vi "Capture@ImageSave__Parameter.vi"(1 "ParamterIn":string) -> (0 "ParamterOut":string)   [LabVIEW 2020]
uses:
  MainFrame/Global.vi
panel:
  in  "Message":string(combo)
  out "Image":T1(plugin-control)
  in  "Picture":string(combo)
  in  "CamName":string(combo)
  in  "Confirm":bool
  # "Capture@General $Capture,$Picture(,[[$label]]$Message)"
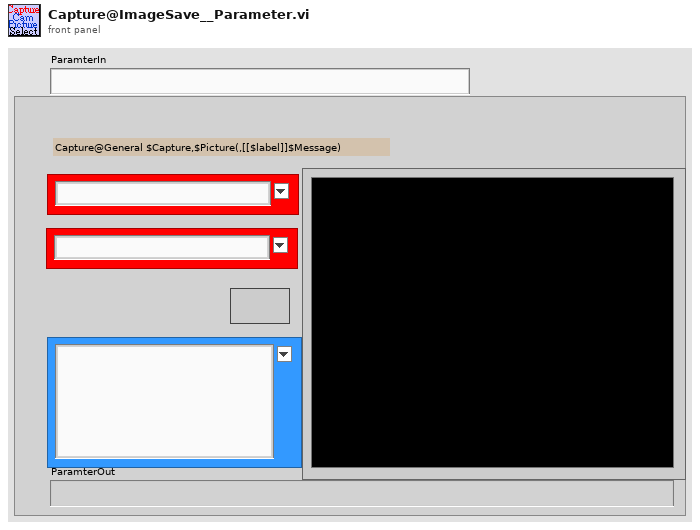
[diagram p1: front panel]
types:
  T1 = typedef "IMAQ Image.ctl" = refnum<image>
  T2 = typedef "Image Type" = u32
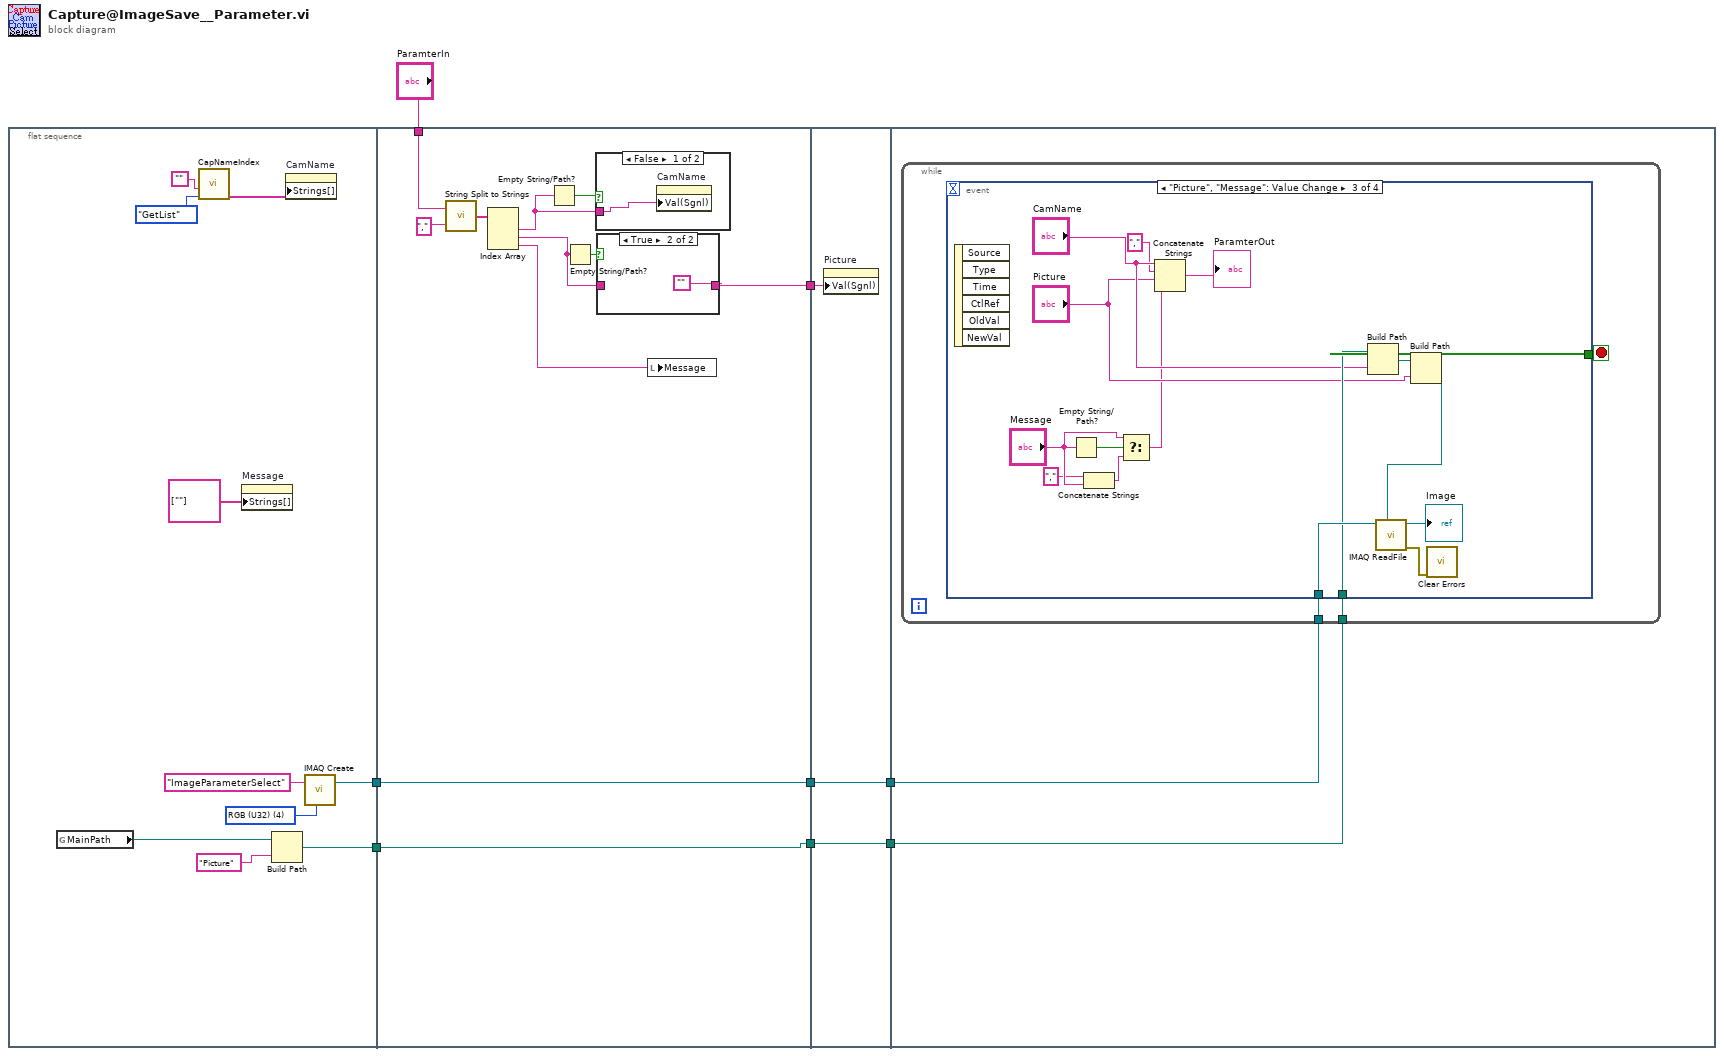
[diagram p0: block diagram]
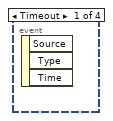
[diagram p4: hidden frame]
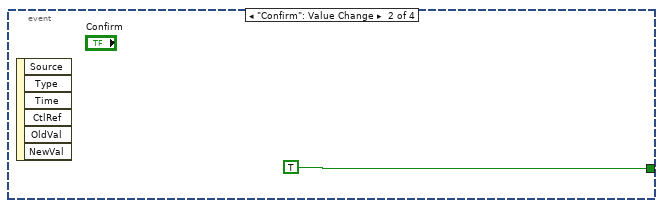
[diagram p5: hidden frame]
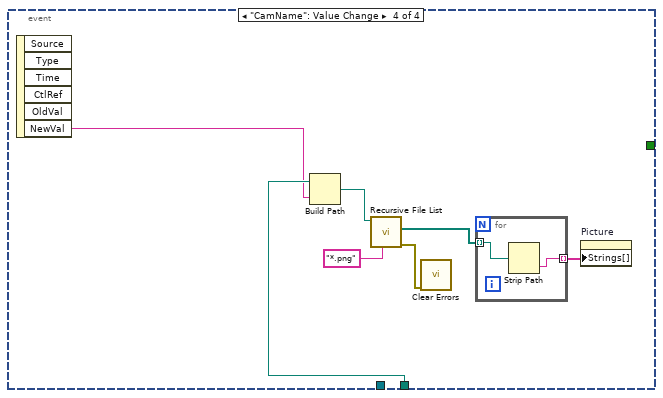
[diagram p6: hidden frame]
diagram:
  n1 = flat-sequence {
    tunnel: [w14] -> w7
    tunnel: [w12] -> w2
    tunnel: "ParamterIn" -> [w27]
    tunnel: w7 -> [w23]
    tunnel: [w23] -> w6
    tunnel: [w21] -> w3
    tunnel: w2 -> [w21]
    tunnel: [w20] -> w1
    tunnel: w6 -> [w35]
    tunnel: [w35] -> w5
    tunnel: [w34] -> w4
    tunnel: w3 -> [w34]
    tunnel: w1 -> [w33]
    tunnel: w5 -> [w37]
    tunnel: w4 -> [w36]
    frame #0 {
      w10 = T2 4 items=["Grayscale (U8)", "Grayscale (I16)", "Grayscale (SGL)", "Complex (CSG)", "RGB (U32)", "HSL (U32)", "RGB (U64)", "Grayscale (U16)"] ("Image Type")
      n2 = global read "Global.vi" "MainPath"() -> (w11:path)
      n3 = call "CapNameIndex.vi"("OP"=enum16{"AddCam", "GetIndex", "Init", "GetList"}."GetList", "CamName"="") -> ("DeviceList"=w17:string[])  [unwired: 2 in, 3 out]
      n4 = property on="Message" class="CmbBox"("Strings[]"=string[] [""] ("Strings []")) -> ()  [unwired: 2 in, 2 out]
      n5 = Build Path(base path=w11, name or relative path="Picture") -> (appended path=w12:path)
      n6 = property on="CamName" class="CmbBox"("Strings[]"=w17) -> ()  [unwired: 2 in, 2 out]
      n7 = call "IMAQ Create"("Image Name"="ImageParameterSelect", "Image Type"=w10) -> ("New Image"=w14:T1)  [unwired: 3 in, 1 out]
    }
    frame #1 {
      n8 = call "String Split to Strings.vi"("search string/char (-)"=",", "String"=w27) -> ("Array"=w29:string[])
      n9 = Index Array(array=w29) -> (element #1=w22:string, element #2=w24:string, element #3=w19:string)  [unwired: 3 in]
      n10 = Empty String/Path?(string/path=w22) -> (empty?=w26:bool)
      n11 = Empty String/Path?(string/path=w24) -> (empty?=w25:bool)
      n12 = case shown="False" w26 {
        tunnel: w22 -> [w32 _]
        frame False {
          n13 = property on="CamName" class="CmbBox"("Val(Sgnl)"=w32) -> ()  [unwired: 2 in, 2 out]
        }
        frame True {
        }
      }
      n14 = case shown="True" w25 {
        tunnel: [w30 ""] -> w20
        tunnel: w24 -> [w30 _]
        frame False {
        }
        frame True {
        }
      }
      n15 = local write "Message"(w19) -> ()
    }
    frame #2 {
      n16 = property on="Picture" class="CmbBox"("Val(Sgnl)"=w33) -> ()  [unwired: 2 in, 2 out]
    }
    frame #3 {
      n17 = while {
        tunnel: w37 -> [w39]
        tunnel: w36 -> [w38]
        stop <- w40 stop-if-true
        n18 = event shown="[2] \"Picture\", \"Message\": Value Change" {
          selector: _ -> [_ _ _ _]
          dyn-events: _ -> [_ _ _ _]
          timeout: _ -> [_ _ _ _]
          tunnel: [_ TRUE _ _] -> w40
          tunnel: w39 -> [_ _ w55 _]
          tunnel: w38 -> [_ _ w54 w60]
          event Timeout {
            n19 = event-data() -> ()  [unwired: 1 in, 3 out]
          }
          event "Confirm": Value Change {
            n20 = event-data() -> ()  [unwired: 1 in, 6 out]
          }
          event "Picture", "Message": Value Change {
            n21 = event-data() -> ()  [unwired: 1 in, 6 out]
            n22 = Empty String/Path?(string/path="Message") -> (empty?=w46:bool)
            n23 = Concatenate Strings("," ("string"), "Message") -> (w45:string)
            n24 = Select(t="Message", s=w46, f=w45) -> (s? t:f=w42:string)
            n25 = Concatenate Strings("CamName", "," ("string"), "Picture", w42) -> (→"ParamterOut":string)
            n26 = Build Path(base path=w54, name or relative path="CamName") -> (appended path=w52:path)
            n27 = Build Path(base path=w52, name or relative path="Picture") -> (appended path=w50:path)
            n28 = call "IMAQ ReadFile"("File Path"=w50, "Image"=w55) -> ("error out"=w49:errorcluster, "Image Out"=→"Image":T1)  [unwired: 5 in, 3 out]
            n29 = call <vilib>:"Clear Errors.vi"("error in (no error)"=w49) -> ()  [unwired: 5 in, 2 out]
          }
          event "CamName": Value Change {
            n30 = event-data() -> ("NewVal"=w59:string)  [unwired: 1 in, 5 out]
            n31 = Build Path(base path=w60, name or relative path=w59) -> (appended path=w58:path)
            n32 = call <vilib>:"Recursive File List.vi"("pattern"="*.png", "Folder Path"=w58) -> ("error out"=w57:errorcluster, "All Files in Dir"=w62:path[])  [unwired: 5 in, 3 out]
            n33 = call <vilib>:"Clear Errors.vi"("error in (no error)"=w57) -> ()  [unwired: 5 in, 2 out]
            n34 = for {
              tunnel: w62 -> [w65] mode=indexing
              tunnel: [w64] -> w63 mode=indexing
              n35 = Strip Path(path=w65) -> (name=w64:string)  [unwired: 1 out]
            }
            n36 = property on="Picture" class="CmbBox"("Strings[]"=w63) -> ()  [unwired: 2 in, 2 out]
          }
        }
      }
    }
  }
